vi "2100-Test-HV Sweep.vi"() -> ()   [LabVIEW 2013]
uses:
  <vilib>/NI_TestStand_SemiconductorModule/NI_TestStand_Semiconductor_Module.lvlibp
  <vilib>/NI_TestStand_SemiconductorModule/NI_TestStand_Semiconductor_Module.lvlibp/PinMap/DC Power/PinsToNIDCPowerSessions.vi
  Controls/USID.ctl
  <vilib>/NI_TestStand_SemiconductorModule/NI_TestStand_Semiconductor_Module.lvlibp/PinMap/General/SemiconductorModuleContext.ctl
panel:
  out "Measurements":dbl[][](array[numeric])
  out "Error Out":errorcluster
  in  "Error In":errorcluster
  in  "Semiconductor Module Context":T1
  in  "All_Scripts":string[][](array[string])
  in  "Pins":string[](array[string])=["CLK", "SDA"]
  in  "USID":T2 max=15
  in  "Test Name":string="IVIOKGD"
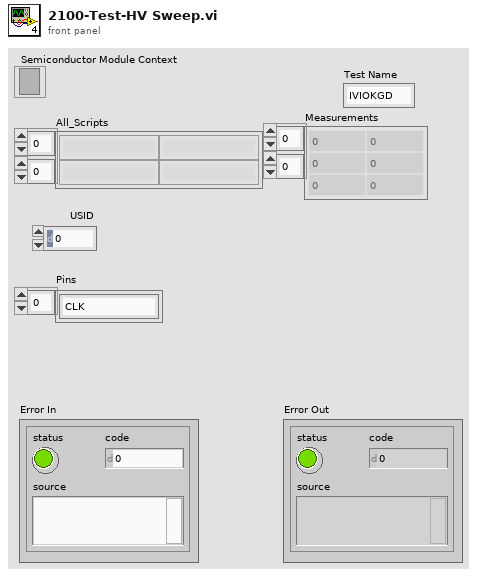
[diagram p1: front panel]
types:
  T1 = typedef "NI_TestStand_Semiconductor_Module.lvlibp/SemiconductorModuleContext.ctl" = refnum<k7>
  T2 = typedef "USID.ctl" = u8
  T3 = typedef "Reg_Address_Data.ctl" = cluster{"Address":u8, "Data":u8}
  T4 = typedef "Script Functions_Array.ctl" = enum16{"Reg_Write", "Bit_Write", "Delay", "Read"}[]
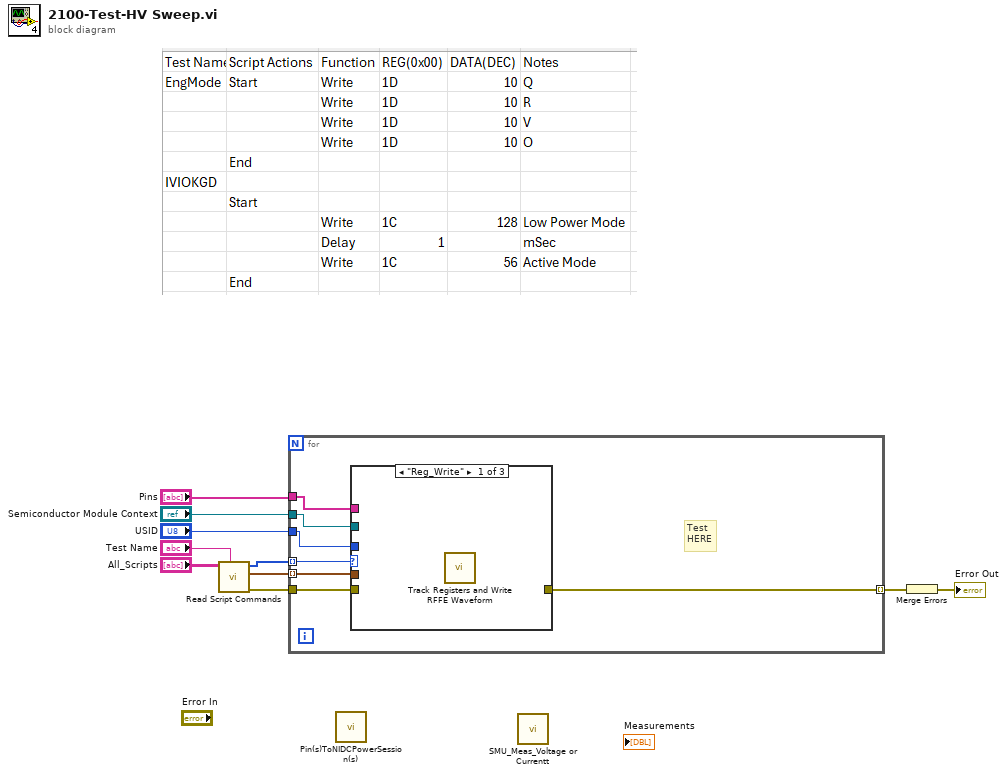
[diagram p0: block diagram]
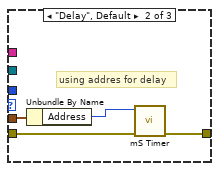
[diagram p2: hidden frame]
diagram:
  n1 = call "Read Script Commands.vi"("Test Name"="Test Name", "All_Scripts"="All_Scripts") -> ("Error Out"=w5:errorcluster, "Script_Data"=w6:T3[], "Script_Functions"=w7:T4)  [unwired: 7 in]
  n2 = for {
    tunnel: "USID" -> [w14]
    tunnel: w7 -> [w17] mode=indexing
    tunnel: w6 -> [w16] mode=indexing
    tunnel: w5 -> [w15]
    tunnel: "Semiconductor Module Context" -> [w13]
    tunnel: "Pins" -> [w12]
    tunnel: [w11] -> w2 mode=indexing
    # "Test \nHERE"
    n3 = case shown="\"Reg_Write\"" w17 {
      tunnel: w16 -> [_ w20 _]
      tunnel: w15 -> [_ w21 w22]
      tunnel: w14 -> [_ _ _]
      tunnel: w13 -> [_ _ _]
      tunnel: w12 -> [_ _ _]
      tunnel: [_ w18 w22] -> w11
      frame "Reg_Write" {
        n4 = call "Track Registers and Write RFFE Waveform.vi"() -> ()  [unwired: 17 in, 3 out]
      }
      frame "Delay", Default {
        # "using addres for delay"
        n5 = Unbundle By Name(w20) -> ("Address"=w19:u8)
        n6 = call "mS Timer.vi"("Error In"=w21, "Delay(S)"=w19) -> ("Error Out"=w18:errorcluster)  [unwired: 9 in]
      }
      frame "Read" {
      }
    }
  }
  n7 = call-poly <vilib>:"Pin(s)ToNIDCPowerSession(s).vi"() -> ()  [unwired: 7 in, 5 out]
  n8 = call "SMU_Meas_Voltage or Currentt.vi"() -> ()  [unwired: 9 in, 3 out]
  n9 = Merge Errors(w2) -> (→"Error Out":errorcluster)
